vi "Dynamic Call VI.vi"(6 "VI路径":path, 8 "错误输入（无错误）":errorcluster, 11 "异步调用线程簇":T1) -> (0 "错误输出":errorcluster, 3 "响应报文主体":string)   [LabVIEW 2019, in "HTTP Server.lvlib"]
uses:
  HTTP Server.lvlib
  Async Thread.ctl
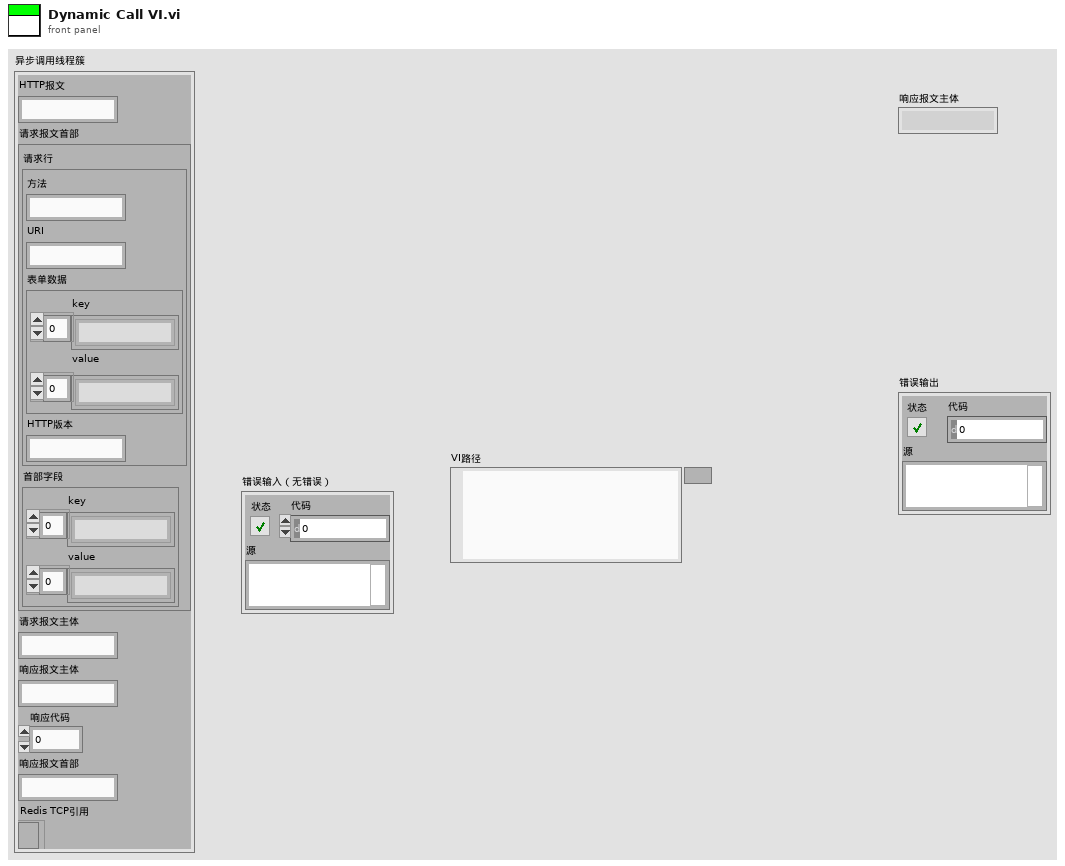
[diagram p1: front panel]
types:
  T1 = typedef "HTTP Server.lvlib/Async Thread.ctl" = cluster{"HTTP报文":string, "请求报文首部":cluster{"请求行":cluster{"方法":string, "URI":string, "表单数据":cluster{"key":string[], "value":string[]}, "HTTP版本":string}, "首部字段":cluster{"key":string[], "value":string[]}}, "请求报文主体":string, "响应报文主体":string, "响应代码":u16, "响应报文首部":string, "Redis TCP引用":refnum<k5>}
  T2 = enum32{"invalid app kind", "Development System", "Run Time System", "Student Edition", "Embedded LabVIEW", "Evaluation", "Custom"}
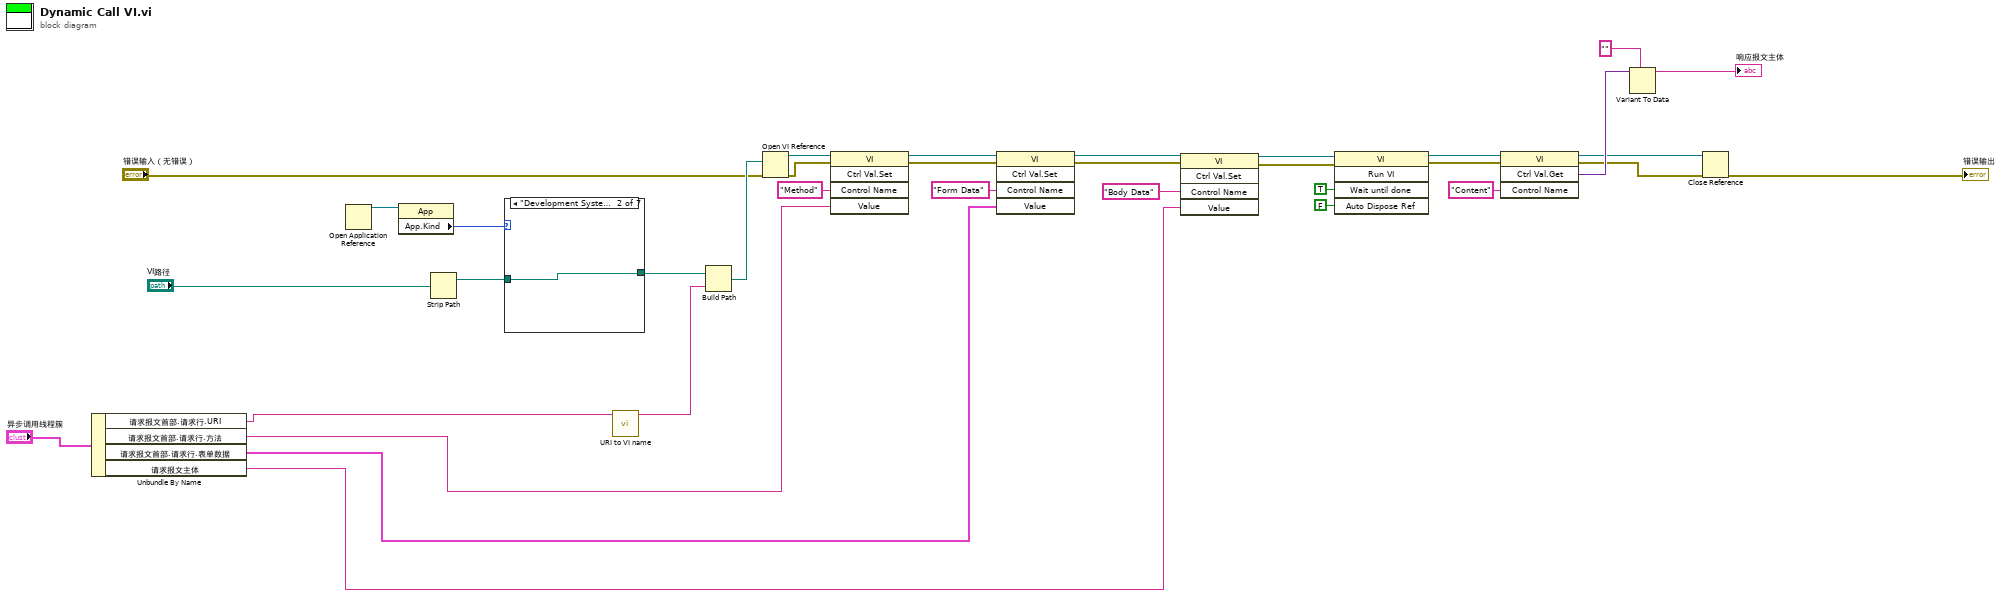
[diagram p0: block diagram]
diagram:
  n1 = Unbundle By Name("异步调用线程簇") -> ("请求报文首部.请求行.URI"=w4:string, "请求报文首部.请求行.方法"=w3:string, "请求报文首部.请求行.表单数据"=w2:cluster{"key":string[], "value":string[]}, "请求报文主体"=w1:string)
  n2 = Open Application Reference() -> (3:w35:refnum<vi>)  [unwired: 4 in, 1 out]
  n3 = property class="App"(reference=w35) -> ("App.Kind"=w34:T2)  [unwired: 1 in, 2 out]
  n4 = Strip Path(path="VI路径") -> (stripped path=w33:path)  [unwired: 1 out]
  n5 = case shown="\"Development System\"" w34 {
    tunnel: w33 -> [w36 w37 w38 w39 w40 w41 w42]
    tunnel: [w36 w37 w38 w39 w40 w41 w42] -> w32
    frame "invalid app kind", Default {
    }
    frame "Development System" {
    }
    frame "Run Time System" {
    }
    frame "Student Edition" {
    }
    frame "Embedded LabVIEW" {
    }
    frame "Evaluation" {
    }
    frame "Custom" {
    }
  }
  n6 = call "URI to VI name.vi"("URI"=w4) -> ("VI name"=w31:string)  [unwired: 10 in]
  n7 = Build Path(base path=w32, name or relative path=w31) -> (appended path=w29:path)
  n8 = Open VI Reference(vi path=w29, error in (no error)="错误输入（无错误）") -> (vi reference=w30:refnum<vi>, error out=w22:errorcluster)  [unwired: 4 in]
  n9 = invoke class="VI" method="Ctrl Val.Set"(reference=w30, error in=w22, "Control Name"="Method" ("控件名"), "Value"=w3) -> (reference out=w14:refnum<vi>, error out=w12:errorcluster)  [unwired: 1 in, 3 out]
  n10 = invoke class="VI" method="Ctrl Val.Set"(reference=w14, error in=w12, "Control Name"="Form Data" ("控件名"), "Value"=w2) -> (reference out=w13:refnum<vi>, error out=w11:errorcluster)  [unwired: 1 in, 3 out]
  n11 = invoke class="VI" method="Ctrl Val.Set"(reference=w13, error in=w11, "Control Name"="Body Data" ("控件名"), "Value"=w1) -> (reference out=w8:refnum<vi>, error out=w7:errorcluster)  [unwired: 1 in, 3 out]
  n12 = invoke class="VI" method="Run VI"(reference=w8, error in=w7, "Wait until done"=TRUE ("结束前等待"), "Auto Dispose Ref"=FALSE ("自动销毁引用")) -> (reference out=w25:refnum<vi>, error out=w23:errorcluster)  [unwired: 1 in, 3 out]
  n13 = invoke class="VI" method="Ctrl Val.Get"(reference=w25, error in=w23, "Control Name"="Content" ("控件名")) -> (reference out=w19:refnum<vi>, error out=w18:errorcluster, "Get Control Value Variant"=w21:variant)  [unwired: 1 in, 1 out]
  n14 = Variant To Data(type="", Variant=w21) -> (data=→"响应报文主体":string)  [unwired: 1 in, 1 out]
  n15 = Close Reference(reference=w19, error in (no error)=w18) -> (error out=→"错误输出":errorcluster)
